vi "Parse Opcode.vi"(8 "error in":errorcluster, 11 "Opcode":string) -> (0 "Error out":errorcluster, 3 "Opcode Array":string[](array[string]))   [LabVIEW 2018, in "Config_Read_BML.lvclass"]
uses:
  Config_Read_BML.lvclass
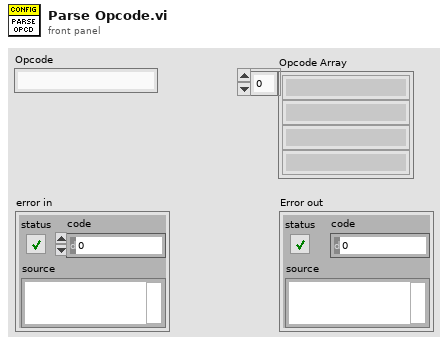
[diagram p1: front panel]
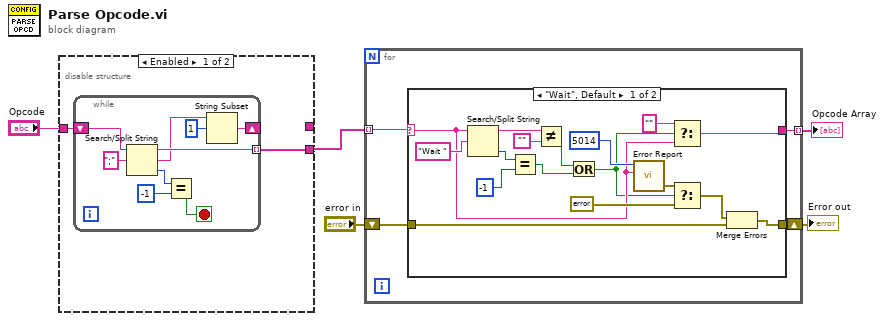
[diagram p0: block diagram]
diagram:
  n1 = disable-structure shown="Enabled" {
    disable-tunnel: "Opcode" -> [w7 w17]
    disable-tunnel: [_ w17] -> _
    disable-tunnel: [w6 _] -> w3
    frame Enabled {
      n2 = while {
        shift-right: [w10] -> _
        shift-left: w7 -> [w15]
        tunnel: [w11] -> w6 mode=indexing
        stop <- w12 stop-if-true
        n3 = Search/Split String(string=w15, search string/char (-)=";") -> (substring before match=w11:string, match + rest of string=w9:string, offset of match=w14:i32)  [unwired: 1 in]
        n4 = Equal?(x=w14, y=-1) -> (x = y?=w12:bool)
        n5 = String Subset(string=w9, offset (0)=1) -> (substring=w10:string)  [unwired: 1 in]
      }
    }
    frame Disabled {
    }
  }
  n6 = for {
    shift-right: [w21] -> w5
    shift-left: "error in" -> [w19]
    tunnel: w3 -> [w20] mode=indexing
    tunnel: [w18] -> w1 mode=indexing
    n7 = case shown="\"Wait\", Default" w20 {
      selector: w20 -> [w27 w40]
      tunnel: [w28 w39] -> w21
      tunnel: [w32 w40] -> w18
      tunnel: w19 -> [w29 w39]
      frame "Wait", Default {
        n8 = Search/Split String(string=w27, search string/char (-)="Wait " ("search string")) -> (substring before match=w26:string, offset of match=w37:i32)  [unwired: 1 in, 1 out]
        n9 = Equal?(x=w37, y=-1) -> (x = y?=w23:bool)
        n10 = Not Equal?(x=w26, y="") -> (x != y?=w24:bool)
        n11 = Or(x=w24, y=w23) -> (x .or. y?=w22:bool)
        n12 = call "Error Report.vi"("Additional info"=w27, "Error Code"=i16 5014) -> ("error out"=w34:errorcluster)  [unwired: 9 in]
        n13 = Select(t="", s=w22, f=w27) -> (s? t:f=w32:string)
        n14 = Select(t=w34, s=w22, f=errorcluster {"status"=FALSE, "code"=0, "source"=""}) -> (s? t:f=w30:errorcluster)
        n15 = Merge Errors(w30, w29) -> (w28:errorcluster)
      }
      frame "", "First", "Last", "Trig", "pulse_signal(event0)" {
      }
    }
  }
  "Error out" <- w5
  "Opcode Array" <- w1
